vi "Comparison By Priority Month Direct.vi"(9 "Starting Month":u32, 10 "Person B":T1={"ID"=0, "Family Name"="Doe", "Given Name"="John", "Birth Date"=timestamp(3533142714.9178333 s since 1904-01-01)} {"Birth Date" format="%<%Y/%b/%d>T"}, 11 "Person A":T1={"ID"=0, "Family Name"="Smith", "Given Name"="John", "Birth Date"=timestamp(3533056306.0488334 s since 1904-01-01)} {"Birth Date" format="%<%Y/%b/%d>T"}) -> (3 "Swap?":bool)   [LabVIEW 2023]
doc: "This VI says that the two values should swap if Person A has a later birthday. If they have the same birthday, then they should swap if Person A has an alphabetically later name than Person B, checking last name first and then first name."
uses:
  Person Information.ctl
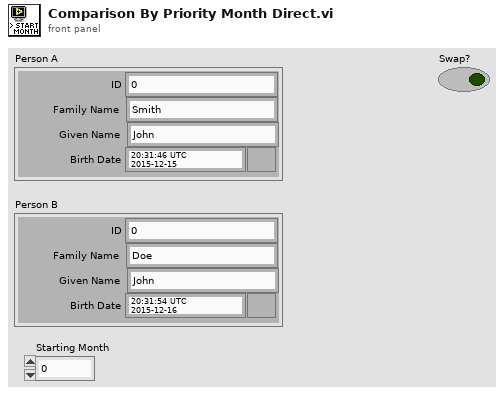
[diagram p1: front panel]
types:
  T1 = typedef "Person Information.ctl" = cluster{"ID":u32, "Family Name":string, "Given Name":string, "Birth Date":timestamp}
  T2 = typedef "LVDateTimeRec.ctl" = cluster{"fractional second":dbl, "second":i32, "minute":i32, "hour":i32, "day of month":i32, "month":i32, "year":i32, "day of week":i32, "day of year":i32, "DST":i32}
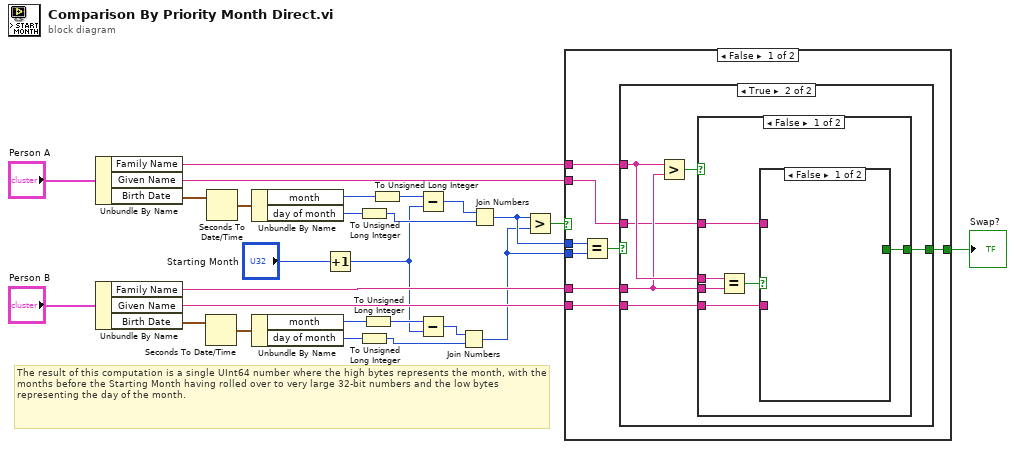
[diagram p0: block diagram]
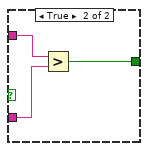
[diagram p3: hidden frame]
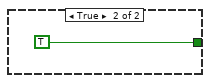
[diagram p4: hidden frame]
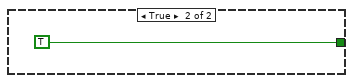
[diagram p5: hidden frame]
diagram:
  # "The result of this computation is a single UInt64 number where the high bytes represents the month, with the months before the Starting Month having rolled over to very large 32-bit numbers and the low bytes representing the day of the month."
  n1 = Unbundle By Name("Person A") -> ("Family Name"=w22:string, "Given Name"=w20:string, "Birth Date"=w18:timestamp)
  n2 = Unbundle By Name("Person B") -> ("Family Name"=w21:string, "Given Name"=w19:string, "Birth Date"=w17:timestamp)
  n3 = Seconds To Date/Time(time stamp (now)=w17) -> (date time rec=w15:T2)  [unwired: 1 in]
  n4 = Seconds To Date/Time(time stamp (now)=w18) -> (date time rec=w16:T2)  [unwired: 1 in]
  n5 = Unbundle By Name(w16) -> ("month"=w14:i32, "day of month"=w12:i32)
  n6 = Unbundle By Name(w15) -> ("month"=w10:i32, "day of month"=w8:i32)
  n7 = Increment(x="Starting Month") -> (x+1=w1:u32)
  n8 = To Unsigned Long Integer(number=w12) -> (unsigned 32bit integer=w6:u32)
  n9 = To Unsigned Long Integer(number=w8) -> (unsigned 32bit integer=w4:u32)
  n10 = To Unsigned Long Integer(number=w10) -> (unsigned 32bit integer=w9:u32)
  n11 = To Unsigned Long Integer(number=w14) -> (unsigned 32bit integer=w13:u32)
  n12 = Subtract(x=w13, y=w1) -> (x-y=w7:u32)
  n13 = Subtract(x=w9, y=w1) -> (x-y=w5:u32)
  n14 = Join Numbers(hi=w5, lo=w4) -> ((hi.lo)=w2:u64)
  n15 = Join Numbers(hi=w7, lo=w6) -> ((hi.lo)=w3:u64)
  n16 = Greater?(x=w3, y=w2) -> (0:w23:bool)
  n17 = case shown="False" w23 {
    tunnel: [w31 TRUE] -> w24
    tunnel: w22 -> [w33 _]
    tunnel: w21 -> [w32 _]
    tunnel: w20 -> [w30 _]
    tunnel: w19 -> [w29 _]
    tunnel: w3 -> [w28 _]
    tunnel: w2 -> [w27 _]
    frame False {
      n18 = Equal?(x=w28, y=w27) -> (x = y?=w34:bool)
      n19 = case shown="True" w34 {
        tunnel: w33 -> [_ w38]
        tunnel: w32 -> [_ w37]
        tunnel: [_ w39] -> w31
        tunnel: w30 -> [_ w36]
        tunnel: w29 -> [_ w35]
        frame False {
        }
        frame True {
          n20 = Greater?(x=w38, y=w37) -> (0:w40:bool)
          n21 = case shown="False" w40 {
            tunnel: [w41 TRUE] -> w39
            tunnel: w38 -> [w46 _]
            tunnel: w37 -> [w45 _]
            tunnel: w36 -> [w43 _]
            tunnel: w35 -> [w42 _]
            frame False {
              n22 = Equal?(x=w46, y=w45) -> (x = y?=w44:bool)
              n23 = case shown="False" w44 {
                tunnel: w43 -> [_ w49]
                tunnel: w42 -> [_ w48]
                tunnel: [_ w47] -> w41
                frame False {
                }
                frame True {
                  n24 = Greater?(x=w49, y=w48) -> (0:w47:bool)
                }
              }
            }
            frame True {
            }
          }
        }
      }
    }
    frame True {
    }
  }
  "Swap?" <- w24
